vi "VerifyVIsNotBroken.vi"() -> ()   [LabVIEW 2020]
panel:
  out "result":string
  out "pass":bool
  out "error out":errorcluster
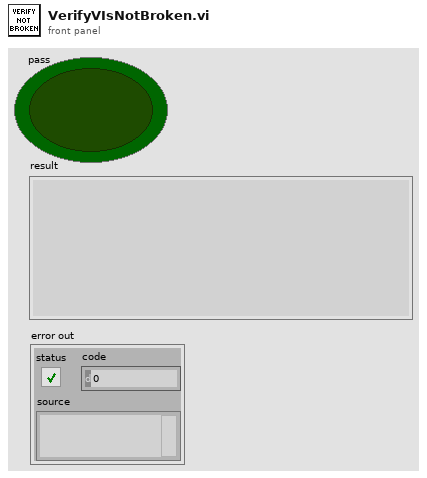
[diagram p1: front panel]
types:
  T1 = enum32{"Bad", "Idle", "Run top level", "Running"}
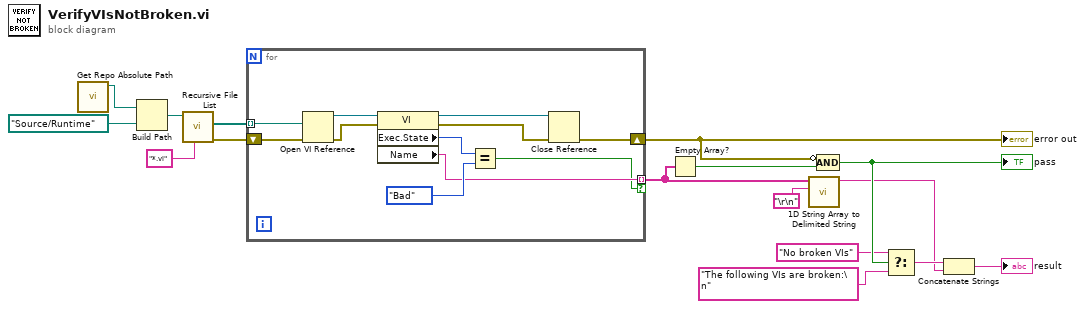
[diagram p0: block diagram]
diagram:
  n1 = call "Get Repo Absolute Path.vi"() -> ("repo path"=w4:path)  [unwired: 11 in]
  n2 = Build Path(base path=w4, name or relative path=path "Source/Runtime") -> (appended path=w3:path)
  n3 = call <vilib>:"Recursive File List.vi"("pattern"="*.vi", "Folder Path"=w3) -> ("error out"=w6:errorcluster, "All Files in Dir"=w1:path[])  [unwired: 5 in, 3 out]
  n4 = for {
    tunnel: w1 -> [w21] mode=indexing
    shift-right: [w27] -> w13
    shift-left: w6 -> [w22]
    tunnel: [w18] -> w15 mode=indexing if=w17
    n5 = Open VI Reference(vi path=w21, error in (no error)=w22) -> (vi reference=w25:refnum<vi>, error out=w26:errorcluster)  [unwired: 4 in]
    n6 = property class="VI"(reference=w25, error in=w26) -> (reference out=w24:refnum<vi>, error out=w23:errorcluster, "Exec.State"=w20:T1, "Name"=w18:string)
    n7 = Equal?(x=w20, y=T1."Bad") -> (x = y?=w17:bool)
    n8 = Close Reference(reference=w24, error in (no error)=w23) -> (error out=w27:errorcluster)
  }
  "error out" <- w13
  n9 = Empty Array?(array=w15) -> (empty?=w14:bool)
  n10 = call <vilib>:"1D String Array to Delimited String.vi"("delimiter"="\r\n", "string array"=w15) -> ("delimited string"=w8:string)  [unwired: 9 in]
  n11 = Compound Arithmetic op=AND(invert w13, w14) -> (w12:bool)
  "pass" <- w12
  n12 = Select(t="No broken VIs", s=w12, f="The following VIs are broken:\n") -> (s? t:f=w9:string)
  n13 = Concatenate Strings(w9, w8) -> (→"result":string)
